vi "ThreePts_Circumcircle.vi"(2 "V3":dbl[](array[numeric]), 3 "V2":dbl[](array[numeric]), 4 "V1":dbl[](array[numeric])) -> (0 "Radius":dbl, 1 "Circumcenter":dbl[](array[numeric]) format="%.2f")   [LabVIEW 2016, in "ForceField.lvclass"]
uses:
  ForceField.lvclass
  <vilib>/Analysis/baseanly.llb/Real Dot Product.vi
  <vilib>/Analysis/7linalg.llb/Solve Linear Equations (single right hand).vi
  <vilib>/Analysis/_algsub.llb/Real Vector Norm.vi
  <vilib>/Analysis/baseanly.llb/Solve Linear Equations By Cholesky.vi
  <vilib>/Analysis/baseanly.llb/Real Matrix to Compact Array.vi
  <vilib>/Analysis/baseanly.llb/Real Compact Tri-Matrix Linear Eqs.vi
  <vilib>/Analysis/coordinate.llb/Cross Product.vi
  <vilib>/Analysis/7linalg.llb/Solve Linear Eqs (General).vi
  <vilib>/Analysis/7linalg.llb/Solve Linear Eqs (Gen, single right hand).vi
  <vilib>/Analysis/NI_AALBase.lvlib
  <vilib>/Analysis/NI_AALPro.lvlib
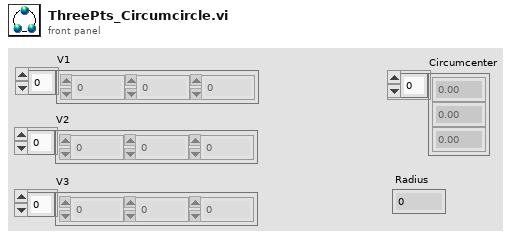
[diagram p1: front panel]
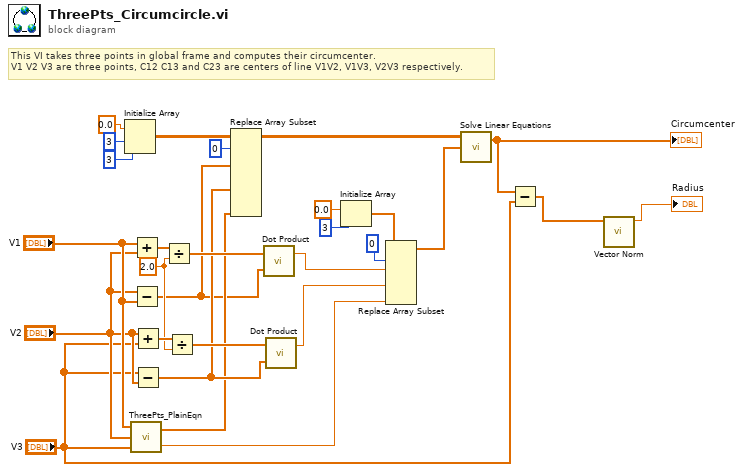
[diagram p0: block diagram]
diagram:
  w26 = 2.0
  # "This VI takes three points in global frame and computes their circumcenter.\nV1 V2 V3 are three points, C12 C13 and C23 are centers of line V1V2, V1V3, V2V3 respectively."
  n1 = Initialize Array(0.0 ("element"), 3 ("dimension size"), 3 ("dimension size")) -> (w21:dbl[][])
  n2 = call "ThreePts_PlainEqn.vi"("V3"="V3", "V2"="V2", "V1"="V1") -> ("D"=w8:dbl, "Normal Vector (A B C)"=w9:dbl[])
  n3 = Add(x="V1", y="V2") -> (x+y=w28:dbl[])
  n4 = Subtract(x="V2", y="V1") -> (x-y=w5:dbl[])
  n5 = Add(x="V2", y="V3") -> (x+y=w27:dbl[])
  n6 = Subtract(x="V3", y="V2") -> (x-y=w18:dbl[])
  n7 = Divide(x=w28, y=w26) -> (x/y=w19:dbl[])
  n8 = Divide(x=w27, y=w26) -> (x/y=w25:dbl[])
  n9 = Replace Array Subset(array=w21, new element #1=w5, index (row) #1=0 ("index (row)"), new element #2=w18, new element #3=w9) -> (w7:dbl[][])  [unwired: 5 in]
  n10 = call-poly <vilib>:"Dot Product.vi"("Y Vector"=w5, "X Vector"=w19) -> ("X * Y"=w13:dbl)  [unwired: 1 out]
  n11 = call-poly <vilib>:"Dot Product.vi"("Y Vector"=w18, "X Vector"=w25) -> ("X * Y"=w12:dbl)  [unwired: 1 out]
  n12 = Initialize Array(0.0 ("element"), 3 ("dimension size")) -> (w15:dbl[])
  n13 = Replace Array Subset(array=w15, new element #1=w13, index #1=0 ("index"), new element #2=w12, new element #3=w8) -> (w6:dbl[])  [unwired: 2 in]
  n14 = call-poly <vilib>:"Solve Linear Equations.vi"("Known Vector"=w6, "Input Matrix"=w7) -> ("Solution Vector"=w4:dbl[])  [unwired: 1 in, 1 out]
  "Circumcenter" <- w4
  n15 = Subtract(x=w4, y="V3") -> (x-y=w2:dbl[])
  n16 = call-poly <vilib>:"Vector Norm.vi"("Input Vector"=w2) -> ("norm"=→"Radius":dbl)  [unwired: 9 in, 1 out]
